vi "HideUnusedControls.vi"(10 "last used index":i32, 11 "control array":refnum<vi>[](array[refnum])) -> ()   [LabVIEW 2009, in "NavScreen.lvlib"]
uses:
  NavScreen.lvlib
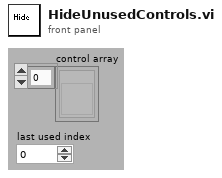
[diagram p1: front panel]
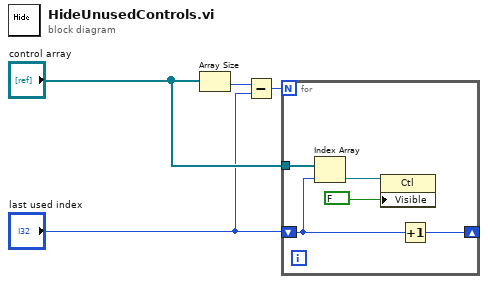
[diagram p0: block diagram]
diagram:
  n1 = Array Size(array="control array") -> (size(s)=w4:i32)
  n2 = Subtract(x=w4, y="last used index") -> (x-y=w3:i32)
  n3 = for {
    N: w3 -> [_]
    shift-right: [w6] -> _
    shift-left: "last used index" -> [w7]
    tunnel: "control array" -> [w9]
    n4 = Index Array(array=w9, index=w7) -> (element=w8:refnum<vi>)
    n5 = property class="Ctl"(reference=w8, "Visible"=FALSE) -> ()  [unwired: 1 in, 2 out]
    n6 = Increment(x=w7) -> (x+1=w6:i32)
  }
